vi "SetLFLockIn.vi"(8 "error in":T4, 11 "LF Lockin Cluster":T1={"Amplitude"=-inf, "Integration Time"=-inf, "Frequency"=-inf, "Output Connector"=-2147483648, "Sensitivity"=-inf, "Input Connector"=-2147483648, "Phase Shift"=-2147483600.0} {"Phase Shift" format="%#_g deg"; "Input Connector" items=["[read only]"=-2147483648, "ADC 1"=0, "ADC 2"=1, "ADC 3"=2, "ADC 4"=3, "ADC 5"=4, "ADC 6"=5, "SPM Z out"=9, "SPM Z out inv"=18, "AFM Signal"=12, "AFM df"=8, "AFM Aexc"=7, "AFM Aosc"=13, "AFM Phase"=14, "Lockin Ampl"=16, "Lockin Phase"=17]; "Sensitivity" format="%#_g V"; "Output Connector" items=["[read only]"=-2147483648, "Off"=0, "DAC 1"=1, "DAC 2"=2, "DAC 1 + DAC 2"=3]; "Frequency" format="%#_g kHz"; "Integration Time" format="%#_g µs"; "Amplitude" format="%#_g V"}) -> (0 "error out":T4, 3 "Output Cluster":T1={"Amplitude"=-inf, "Integration Time"=-inf, "Frequency"=-inf, "Output Connector"=-2147483648, "Sensitivity"=-inf, "Input Connector"=-2147483648, "Phase Shift"=-2147483600.0} {"Phase Shift" format="%#_g deg"; "Input Connector" items=["[read only]"=-2147483648, "ADC 1"=0, "ADC 2"=1, "ADC 3"=2, "ADC 4"=3, "ADC 5"=4, "ADC 6"=5, "SPM Z out"=9, "SPM Z out inv"=18, "AFM Signal"=12, "AFM df"=8, "AFM Aexc"=7, "AFM Aosc"=13, "AFM Phase"=14, "Lockin Ampl"=16, "Lockin Phase"=17]; "Sensitivity" format="%#_g V"; "Output Connector" items=["[read only]"=-2147483648, "Off"=0, "DAC 1"=1, "DAC 2"=2, "DAC 1 + DAC 2"=3]; "Frequency" format="%#_g kHz"; "Integration Time" format="%#_g µs"; "Amplitude" format="%#_g V"})   [LabVIEW 2016]
doc: "Sets all parameters relevant to the low frequency lock in. The input cluster contains:\n- Amplitude in V (float) [0 to 10]\n- Frequency in kHz (float) [0 to 20]\n- Sensitivity in V (float) [0 to 10]\n- Phase Shift in deg (float) [0 to 360]\n- Integration Time in us (float) [1 to 163000]\n- Output Connector (integer) [0 -- off; 1 -- DAC1; 2 -- DAC2; 3 -- DAC1+DAC2]\n- Input Connector (integer) [0-5 -- ADC1-6; 7 -- AFM Aexc; 8 -- AFM df; 9 -- SPM Z out; 12 -- AFM Signal; 13 -- AFM Aosc; 14 -- AFM Phase; 16 -- LockIn Ampl; 17 -- LockIn Phase; 18 -- SPM Z out inv] \nBy passing -Inf (float) or -2147483648 (integer) as input values, the corresponding parameter(s) will be read out."
uses:
  Controls/LF-Lockin_Parameters.ctl
  Controls/LF-Lockin-Output-Connector_Selection.ctl
  Controls/LF-Lockin-Input-Connector_Selection.ctl
  Controls/Error_Out.ctl
  Files_ASC500/DLL/ASC500_RemoteControlV27.dll
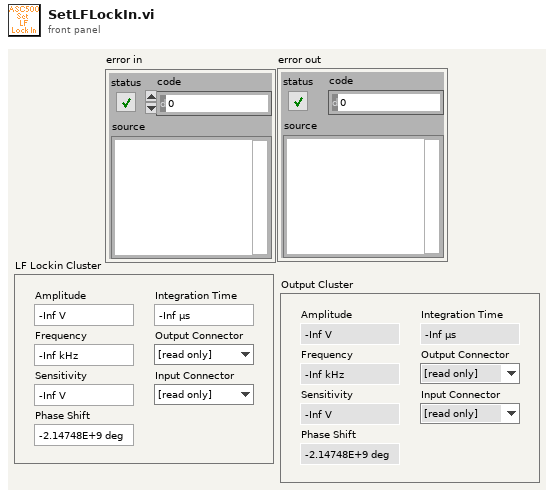
[diagram p1: front panel]
types:
  T1 = typedef "LF-Lockin_Parameters.ctl" = cluster{"Amplitude":sgl, "Integration Time":sgl, "Frequency":sgl, "Output Connector":T2, "Sensitivity":sgl, "Input Connector":T3, "Phase Shift":sgl}
  T2 = typedef "LF-Lockin-Output-Connector_Selection.ctl" = i32
  T3 = typedef "LF-Lockin-Input-Connector_Selection.ctl" = i32
  T4 = typedef "Error_Out.ctl" = errorcluster
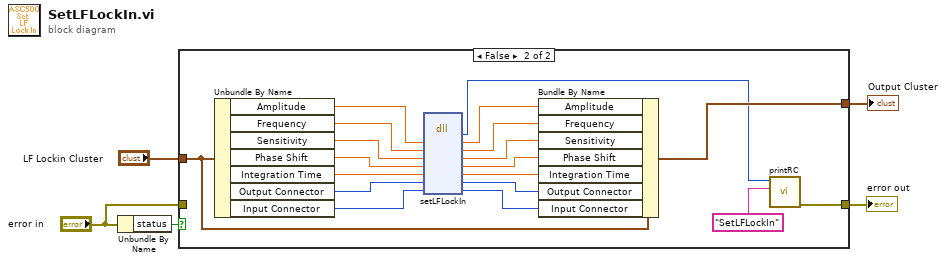
[diagram p0: block diagram]
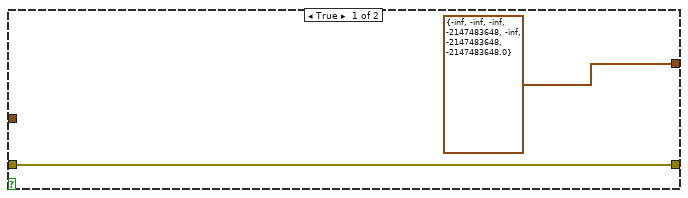
[diagram p2: hidden frame]
diagram:
  n1 = Unbundle By Name("error in") -> ("status"=w5:bool)
  n2 = case shown="False" w5 {
    tunnel: [w6 w10] -> w4
    tunnel: "LF Lockin Cluster" -> [_ w12]
    tunnel: [T1 {"Amplitude"=-inf, "Integration Time"=-inf, "Frequency"=-inf, "Output Connector"=-2147483648, "Sensitivity"=-inf, "Input Connector"=-2147483648, "Phase Shift"=-2147483600.0} ("LF Lockin Cluster") w11] -> w2
    tunnel: "error in" -> [w6 _]
    frame True {
    }
    frame False {
      n3 = Unbundle By Name(w12) -> ("Amplitude"=w26:sgl, "Frequency"=w25:sgl, "Sensitivity"=w24:sgl, "Phase Shift"=w23:sgl, "Integration Time"=w22:sgl, "Output Connector"=w14:T2, "Input Connector"=w13:T3)
      n4 = dll-call lib="G:/SCMOperations/Share/ELE/Produkt Information/ASC500/04 Remote Control/02 development versions/2018Nov06/Files_ASC500/DLL/ASC500_RemoteControlV27.dll" fn="setLFLockIn"("Amplitude"=w26, "Frequency"=w25, "Sensitivity"=w24, "Phase Shift"=w23, "Integration Time"=w22, "Output Connector"=w14, "Input Connector"=w13) -> ("return type"=w9:i32, "Amplitude"=w21:sgl, "Frequency"=w20:sgl, "Sensitivity"=w19:sgl, "Phase Shift"=w18:sgl, "Integration Time"=w17:sgl, "Output Connector"=w16:i32, "Input Connector"=w15:i32)  [unwired: 3 in, 2 out]
      n5 = Bundle By Name(cluster=w12, "Amplitude"=w21, "Frequency"=w20, "Sensitivity"=w19, "Phase Shift"=w18, "Integration Time"=w17, "Output Connector"=w16, "Input Connector"=w15) -> (w11:T1)
      n6 = call "printRC.vi"("additional information"="SetLFLockIn", "RC"=w9) -> ("error out"=w10:T4)  [unwired: 9 in]
    }
  }
  "error out" <- w4
  "Output Cluster" <- w2
